vi "unflattenForceFromXML_Scalar.vi"(8 "error in (no error)":errorcluster, 9 "forceUnitInXML":T1, 10 "xmlString":string, 11 "forceForType":dbl[unit]) -> (0 "error out":errorcluster, 3 "force":dbl[unit])   [LabVIEW 2012, in "UnitsAndXML.lvlib"]
uses:
  <userlib>/Common/UnitsAndXML/UnitsAndXML.lvlib
  <userlib>/Common/UnitsAndXML/FlattenItemWithUnitToXML/FlattenForceToXML/ForceUnit.ctl
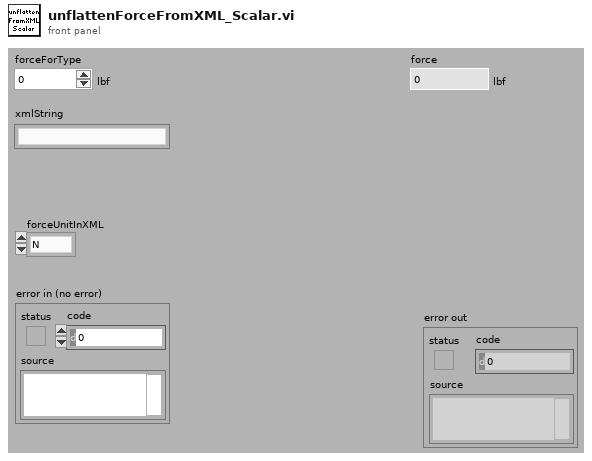
[diagram p1: front panel]
types:
  T1 = typedef "UnitsAndXML.lvlib/ForceUnit.ctl" = enum16{"N", "dyn", "lbf"}
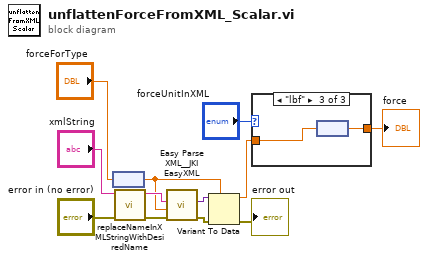
[diagram p0: block diagram]
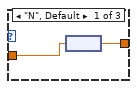
[diagram p2: hidden frame]
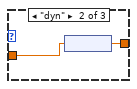
[diagram p3: hidden frame]
diagram:
  n1 = node("forceForType") -> (w7:dbl)
  n2 = call <userlib>:"replaceNameInXMLStringWithDesiredName.vi"("error in"="error in (no error)", "xmlString"="xmlString") -> ("error out"=w1:errorcluster, "revisedXMLString"=w9:string)  [unwired: 8 in]
  n3 = call <vilib>:"Easy Parse XML__JKI EasyXML.vi"("error in (no error)"=w1, "LabVIEW Data (Type)"=w7, "XML String"=w9) -> ("error out"=w4:errorcluster, "LabVIEW Data"=w11:variant)  [unwired: 7 in]
  n4 = Variant To Data(error in=w4, type=w7, Variant=w11) -> (data=w6:dbl, error out=→"error out":errorcluster)
  n5 = case shown="\"lbf\"" "forceUnitInXML" {
    tunnel: w6 -> [w14 w16 w18]
    tunnel: [w13 w15 w17] -> w5
    frame "N", Default {
      n6 = node(w14) -> (w13:dbl[unit])
    }
    frame "dyn" {
      n7 = node(w16) -> (w15:dbl[unit])
    }
    frame "lbf" {
      n8 = node(w18) -> (w17:dbl[unit])
    }
  }
  "force" <- w5
